vi "IMS Stepper V2.vi"() -> ()   [LabVIEW 2018]
doc: "Use this template to build a producer/consumer design pattern with events to produce queue items. Use this design pattern instead of the User Interface Event Handler pattern for user interfaces when you want to execute code asynchronously in response to an event without slowing the user interface responsiveness."
uses:
  stepper motor state.ctl
  stepper graphics internal event.ctl
  stepper graphics action.ctl
  stepper graphics internal state.ctl
  publisher action.ctl
  slider action.ctl
panel:
  in  "Tab Control":enum32{"main", "init&stuff", "ignore"}(tab)
  in  "stepper state":T1=enum."stopped"
  in  "set angle":dbl(slide)=-18.244680851063833 scale=-95.0..95.0 scale format="%^#6_6g"
  in  "XY Graph":cluster{dbl[], dbl[]}[](graph)=[{[-0.2849184585575504, -0.22366098996767705, -0.16240352137780373, -0.10114605278793037, -0.03988858419805705, 0.02136888439181628, 0.08262635298168963, 0.14388382157156293, 0.20514129016143628, 0.2663987587513096, 0.32765622734118294, 0.3889136959310563, 0.45017116452092965, 0.511428633110803, 0.5726861017006762, 0.6339435702905496, 0.695201038880423, 0.7564585074702963, 0.8177159760601695, 0.878973444650043], [0.09392269147117449, 0.07372931280487197, 0.053535934138569455, 0.03334255547226694, 0.013149176805964419, -0.007044201860338106, -0.027237580526640617, -0.04743095919294313, -0.06762433785924565, -0.08781771652554818, -0.1080110951918507, -0.1282044738581532, -0.14839785252445573, -0.16859123119075825, -0.18878460985706075, -0.2089779885233633, -0.2291713671896658, -0.2493647458559683, -0.26955812452227085, -0.28975150318857334]}, {[0.02614672282429747, 0.020525177417073513, 0.014903632009849559, 0.0092820866026256, 0.003660541195401646, -0.0019610042118223085, -0.00758254961904627, -0.013204095026270225, -0.01882564043349418, -0.024447185840718134, -0.03006873124794209, -0.03569027665516605, -0.04131182206239001, -0.04693336746961396, -0.05255491287683792, -0.05817645828406187, -0.06379800369128583, -0.06941954909850978, -0.07504109450573374, -0.08066263991295769], [0.2988584094275236, 0.23460385140060602, 0.17034929337368845, 0.10609473534677089, 0.04184017731985329, -0.022414380707064308, -0.08666893873398185, -0.15092349676089944, -0.21517805478781704, -0.27943261281473464, -0.34368717084165223, -0.40794172886856983, -0.4721962868954873, -0.5364508449224049, -0.6007054029493225, -0.6649599609762401, -0.7292145190031577, -0.7934690770300753, -0.8577236350569929, -0.9219781930839105]}, {[1.0, 0.9980267284282716, 0.9921147013144779, 0.9822872507286887, 0.9685831611286311, 0.9510565162951535, 0.9297764858882513, 0.9048270524660195, 0.8763066800438636, 0.8443279255020151, 0.8090169943749475, 0.7705132427757891, 0.7289686274214116, 0.6845471059286886, 0.6374239897486896, 0.587785252292473, 0.5358267949789965, 0.48175367410171516, 0.42577929156507266, 0.36812455268467786, 0.30901699437494745, 0.24868988716485474, 0.18738131458572452, 0.12533323356430426, 0.0627905195293133, -1.6081428723391245e-16, -0.0627905195293134, -0.12533323356430437, -0.18738131458572482, -0.24868988716485485, -0.30901699437494756, -0.368124552684678, -0.4257792915650727, -0.48175367410171543, -0.5358267949789969, -0.587785252292473, -0.6374239897486897, -0.6845471059286887, -0.7289686274214117, -0.7705132427757894, -0.8090169943749473, -0.8443279255020151, -0.8763066800438636, -0.9048270524660196, -0.9297764858882515, -0.9510565162951536, -0.9685831611286311, -0.9822872507286887, -0.9921147013144779, -0.9980267284282716, -1.0, -0.9980267284282716, -0.9921147013144779, -0.9822872507286886, -0.9685831611286311, -0.9510565162951535, -0.9297764858882512, -0.9048270524660195, -0.8763066800438635, -0.844327925502015, -0.8090169943749472, -0.770513242775789, -0.7289686274214116, -0.6845471059286886, -0.6374239897486895, -0.5877852522924732, -0.5358267949789963, -0.48175367410171527, -0.42577929156507216, -0.3681245526846778, -0.30901699437494756, -0.24868988716485443, -0.18738131458572463, -0.12533323356430373, -0.06279051952931321, -1.836909530733566e-16, 0.06279051952931372, 0.12533323356430423, 0.18738131458572513, 0.24868988716485493, 0.30901699437494723, 0.36812455268467825, 0.4257792915650726, 0.4817536741017157, 0.5358267949789968, 0.5877852522924737, 0.63742398974869, 0.6845471059286886, 0.7289686274214119, 0.7705132427757894, 0.8090169943749478, 0.8443279255020153, 0.8763066800438636, 0.9048270524660197, 0.9297764858882515, 0.9510565162951538, 0.9685831611286312, 0.9822872507286887, 0.9921147013144779, 0.9980267284282716], [0.0, 0.06279051952931337, 0.12533323356430426, 0.18738131458572463, 0.2486898871648548, 0.3090169943749474, 0.368124552684678, 0.4257792915650727, 0.4817536741017153, 0.5358267949789967, 0.5877852522924731, 0.6374239897486897, 0.6845471059286887, 0.7289686274214116, 0.7705132427757893, 0.8090169943749475, 0.8443279255020151, 0.8763066800438637, 0.9048270524660196, 0.9297764858882515, 0.9510565162951535, 0.9685831611286311, 0.9822872507286887, 0.9921147013144779, 0.9980267284282716, 1.0, 0.9980267284282716, 0.9921147013144778, 0.9822872507286886, 0.9685831611286311, 0.9510565162951535, 0.9297764858882513, 0.9048270524660195, 0.8763066800438635, 0.844327925502015, 0.8090169943749475, 0.7705132427757893, 0.7289686274214114, 0.6845471059286885, 0.6374239897486895, 0.5877852522924732, 0.5358267949789967, 0.4817536741017152, 0.4257792915650725, 0.36812455268467775, 0.3090169943749471, 0.24868988716485482, 0.18738131458572457, 0.1253332335643041, 0.06279051952931314, -3.216285744678249e-16, -0.06279051952931335, -0.12533323356430429, -0.18738131458572477, -0.24868988716485502, -0.30901699437494773, -0.3681245526846783, -0.42577929156507266, -0.4817536741017154, -0.5358267949789968, -0.5877852522924734, -0.63742398974869, -0.6845471059286887, -0.7289686274214116, -0.7705132427757894, -0.8090169943749473, -0.8443279255020153, -0.8763066800438636, -0.9048270524660198, -0.9297764858882515, -0.9510565162951535, -0.9685831611286312, -0.9822872507286887, -0.9921147013144779, -0.9980267284282716, -1.0, -0.9980267284282716, -0.9921147013144779, -0.9822872507286886, -0.9685831611286311, -0.9510565162951536, -0.9297764858882512, -0.9048270524660196, -0.8763066800438634, -0.844327925502015, -0.809016994374947, -0.770513242775789, -0.7289686274214116, -0.6845471059286883, -0.6374239897486896, -0.5877852522924726, -0.5358267949789963, -0.4817536741017153, -0.4257792915650722, -0.36812455268467786, -0.3090169943749468, -0.2486898871648545, -0.18738131458572468, -0.1253332335643038, -0.06279051952931326]}, {[0.1, 0.09980267284282716, 0.0992114701314478, 0.09822872507286888, 0.09685831611286311, 0.09510565162951536, 0.09297764858882514, 0.09048270524660196, 0.08763066800438636, 0.08443279255020152, 0.08090169943749476, 0.07705132427757892, 0.07289686274214116, 0.06845471059286887, 0.06374239897486897, 0.05877852522924731, 0.05358267949789966, 0.04817536741017152, 0.042577929156507266, 0.03681245526846779, 0.030901699437494747, 0.024868988716485477, 0.018738131458572452, 0.012533323356430426, 0.006279051952931331, -1.6081428723391246e-17, -0.0062790519529313405, -0.012533323356430438, -0.018738131458572484, -0.024868988716485487, -0.030901699437494757, -0.0368124552684678, -0.04257792915650727, -0.048175367410171546, -0.05358267949789969, -0.05877852522924731, -0.06374239897486898, -0.06845471059286888, -0.07289686274214117, -0.07705132427757894, -0.08090169943749474, -0.08443279255020152, -0.08763066800438636, -0.09048270524660196, -0.09297764858882515, -0.09510565162951537, -0.09685831611286311, -0.09822872507286888, -0.0992114701314478, -0.09980267284282716, -0.1, -0.09980267284282716, -0.0992114701314478, -0.09822872507286887, -0.09685831611286311, -0.09510565162951536, -0.09297764858882512, -0.09048270524660196, -0.08763066800438635, -0.0844327925502015, -0.08090169943749473, -0.07705132427757891, -0.07289686274214116, -0.06845471059286887, -0.06374239897486896, -0.05877852522924733, -0.05358267949789963, -0.04817536741017153, -0.04257792915650722, -0.036812455268467784, -0.030901699437494757, -0.024868988716485445, -0.018738131458572463, -0.012533323356430374, -0.006279051952931321, -1.836909530733566e-17, 0.006279051952931373, 0.012533323356430424, 0.018738131458572515, 0.024868988716485494, 0.030901699437494726, 0.036812455268467825, 0.042577929156507266, 0.048175367410171574, 0.05358267949789968, 0.05877852522924737, 0.063742398974869, 0.06845471059286887, 0.07289686274214119, 0.07705132427757894, 0.08090169943749478, 0.08443279255020153, 0.08763066800438636, 0.09048270524660197, 0.09297764858882515, 0.09510565162951538, 0.09685831611286312, 0.09822872507286888, 0.0992114701314478, 0.09980267284282716], [0.0, 0.006279051952931338, 0.012533323356430426, 0.018738131458572463, 0.02486898871648548, 0.03090169943749474, 0.0368124552684678, 0.04257792915650727, 0.04817536741017153, 0.05358267949789967, 0.058778525229247314, 0.06374239897486898, 0.06845471059286888, 0.07289686274214116, 0.07705132427757894, 0.08090169943749476, 0.08443279255020152, 0.08763066800438638, 0.09048270524660196, 0.09297764858882515, 0.09510565162951536, 0.09685831611286311, 0.09822872507286888, 0.0992114701314478, 0.09980267284282716, 0.1, 0.09980267284282716, 0.09921147013144778, 0.09822872507286887, 0.09685831611286311, 0.09510565162951536, 0.09297764858882514, 0.09048270524660196, 0.08763066800438635, 0.0844327925502015, 0.08090169943749476, 0.07705132427757894, 0.07289686274214115, 0.06845471059286885, 0.06374239897486896, 0.05877852522924733, 0.05358267949789967, 0.048175367410171525, 0.04257792915650725, 0.03681245526846778, 0.030901699437494712, 0.024868988716485484, 0.01873813145857246, 0.01253332335643041, 0.0062790519529313145, -3.216285744678249e-17, -0.006279051952931335, -0.01253332335643043, -0.018738131458572477, -0.024868988716485504, -0.030901699437494774, -0.03681245526846783, -0.042577929156507266, -0.04817536741017154, -0.05358267949789968, -0.05877852522924734, -0.063742398974869, -0.06845471059286888, -0.07289686274214116, -0.07705132427757894, -0.08090169943749474, -0.08443279255020153, -0.08763066800438636, -0.09048270524660199, -0.09297764858882515, -0.09510565162951536, -0.09685831611286312, -0.09822872507286888, -0.0992114701314478, -0.09980267284282716, -0.1, -0.09980267284282716, -0.0992114701314478, -0.09822872507286887, -0.09685831611286311, -0.09510565162951537, -0.09297764858882512, -0.09048270524660196, -0.08763066800438635, -0.0844327925502015, -0.0809016994374947, -0.07705132427757891, -0.07289686274214116, -0.06845471059286883, -0.06374239897486897, -0.05877852522924726, -0.05358267949789963, -0.04817536741017153, -0.042577929156507224, -0.03681245526846779, -0.03090169943749468, -0.02486898871648545, -0.01873813145857247, -0.012533323356430379, -0.006279051952931327]}, {[0.0, 0.0, 0.0, 0.0, 0.0, 0.0, 0.0, 0.0, 0.0, 0.0, 0.0, 0.0, 0.0, 0.0, 0.0, 0.0, 0.0, 0.0, 0.0, 0.0], [1.1, 1.135, 1.1700000000000002, 1.205, 1.24, 1.2750000000000001, 1.31, 1.345, 1.3800000000000001, 1.415, 1.4500000000000002, 1.485, 1.52, 1.5550000000000002, 1.59, 1.625, 1.6600000000000001, 1.695, 1.73, 1.7650000000000001]}, {[6.735334946023075e-17, 6.796565263714194e-17, 6.857795581405312e-17, 6.919025899096432e-17, 6.980256216787551e-17, 7.04148653447867e-17, 7.102716852169788e-17, 7.163947169860908e-17, 7.225177487552027e-17, 7.286407805243145e-17, 7.347638122934264e-17, 7.408868440625383e-17, 7.470098758316503e-17, 7.53132907600762e-17, 7.59255939369874e-17, 7.653789711389858e-17, 7.715020029080977e-17, 7.776250346772096e-17, 7.837480664463216e-17, 7.898710982154334e-17], [1.1, 1.11, 1.12, 1.1300000000000001, 1.1400000000000001, 1.1500000000000001, 1.1600000000000001, 1.1700000000000002, 1.1800000000000002, 1.1900000000000002, 1.2000000000000002, 1.21, 1.22, 1.23, 1.24, 1.25, 1.26, 1.27, 1.28, 1.29]}, {[-0.09587131702242406, -0.09674287444990064, -0.09761443187737723, -0.0984859893048538, -0.0993575467323304, -0.10022910415980697, -0.10110066158728355, -0.10197221901476014, -0.10284377644223672, -0.10371533386971331, -0.10458689129718989, -0.10545844872466646, -0.10633000615214305, -0.10720156357961963, -0.10807312100709622, -0.1089446784345728, -0.10981623586204937, -0.11068779328952597, -0.11155935071700254, -0.11243090814447912], [-1.0958141679009201, -1.1057761148818375, -1.115738061862755, -1.1257000088436726, -1.13566195582459, -1.1456239028055073, -1.1555858497864249, -1.1655477967673424, -1.1755097437482598, -1.1854716907291771, -1.1954336377100947, -1.2053955846910123, -1.2153575316719296, -1.225319478652847, -1.2352814256337645, -1.245243372614682, -1.2552053195955994, -1.2651672665765168, -1.2751292135574344, -1.285091160538352]}]
  out "cur angle":dbl(slide)=-95.0 scale=-95.0..95.0 scale format="%^#6_6g"
  in  "set step !":dbl(slide)=6845.744680851064 min=0.0 max=16000.0 scale=0.0..16500.0 scale format="%^#6_6g"
  out "cur step":dbl(slide) scale=0.0..16500.0
  in  "Go!":bool
  in  "Stop!":bool
  in  "set speed!":i32=2500
  out "Moving..":bool
  out "error out":errorcluster
  out "Current Bottom Position":dbl format="%.4f"
  in  "Move to Bottom Position (deg or in)":dbl=95.83933701824397 format="%.4f"
  in  "Rotator":T2(ring)=enum."System B 50 mm Magnet"
  out "Timeout error":bool
  in  "Exit!":bool
  in  "Instrument Address":refnum<visa-resource-name>="ASRL2::INSTR"
  in  "Set to zero!":bool
  in  "Init!":bool
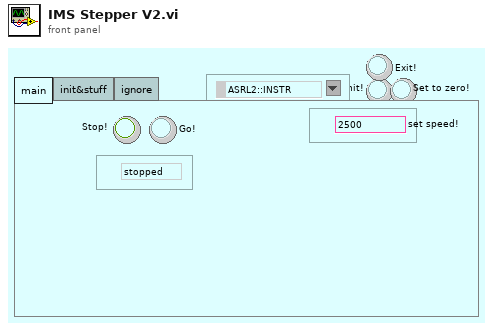
[diagram p1: front panel]
types:
  T1 = typedef "stepper motor state.ctl" = enum16{"moving", "stopped"}
  T2 = enum16{"Dilution Fridge SCM 1", "System A SCM 2", "System B 50 mm Magnet", "He-3 32 mm Magnet", "Portable Dil Fridge Rotator", "Linear Position", "System E Probe 1"}
  T3 = typedef "stepper graphics internal state.ctl" = cluster{"set pos slider":refnum<vi>, "cur angle slider":refnum<vi>, "XY Graph":refnum<vi>, "set angle":dbl, "current angle":dbl, "set angle slider":refnum<vi>, "current pos... slider":refnum<vi>, "current pos":dbl, "set pos":dbl}
  T4 = typedef "stepper graphics action.ctl" = enum16{"--update circle", "set step slider moves", "cursor moves", "current pos changed", "init", "void", "--draw current lie", "--draw set line", "--move current step slider", "--move set step slider", "--draw limit lines", "check", "--move set angle slider", "--move current angle slider", "set angle slider moves", "--move cursor", "set set step", "set current step", "read"}
  T5 = typedef "stepper graphics internal event.ctl" = enum16{"set slider moves", "update scale", "exit", "current positon changed", "stop", "go", "set speed", "set to zero", "sync"}
  T6 = typedef "slider action.ctl" = enum16{"check", "copy range", "set from value", "set from ratio", "set from slider", "read using other slider"}
  T7 = typedef "publisher action.ctl" = enum16{"set", "get"}
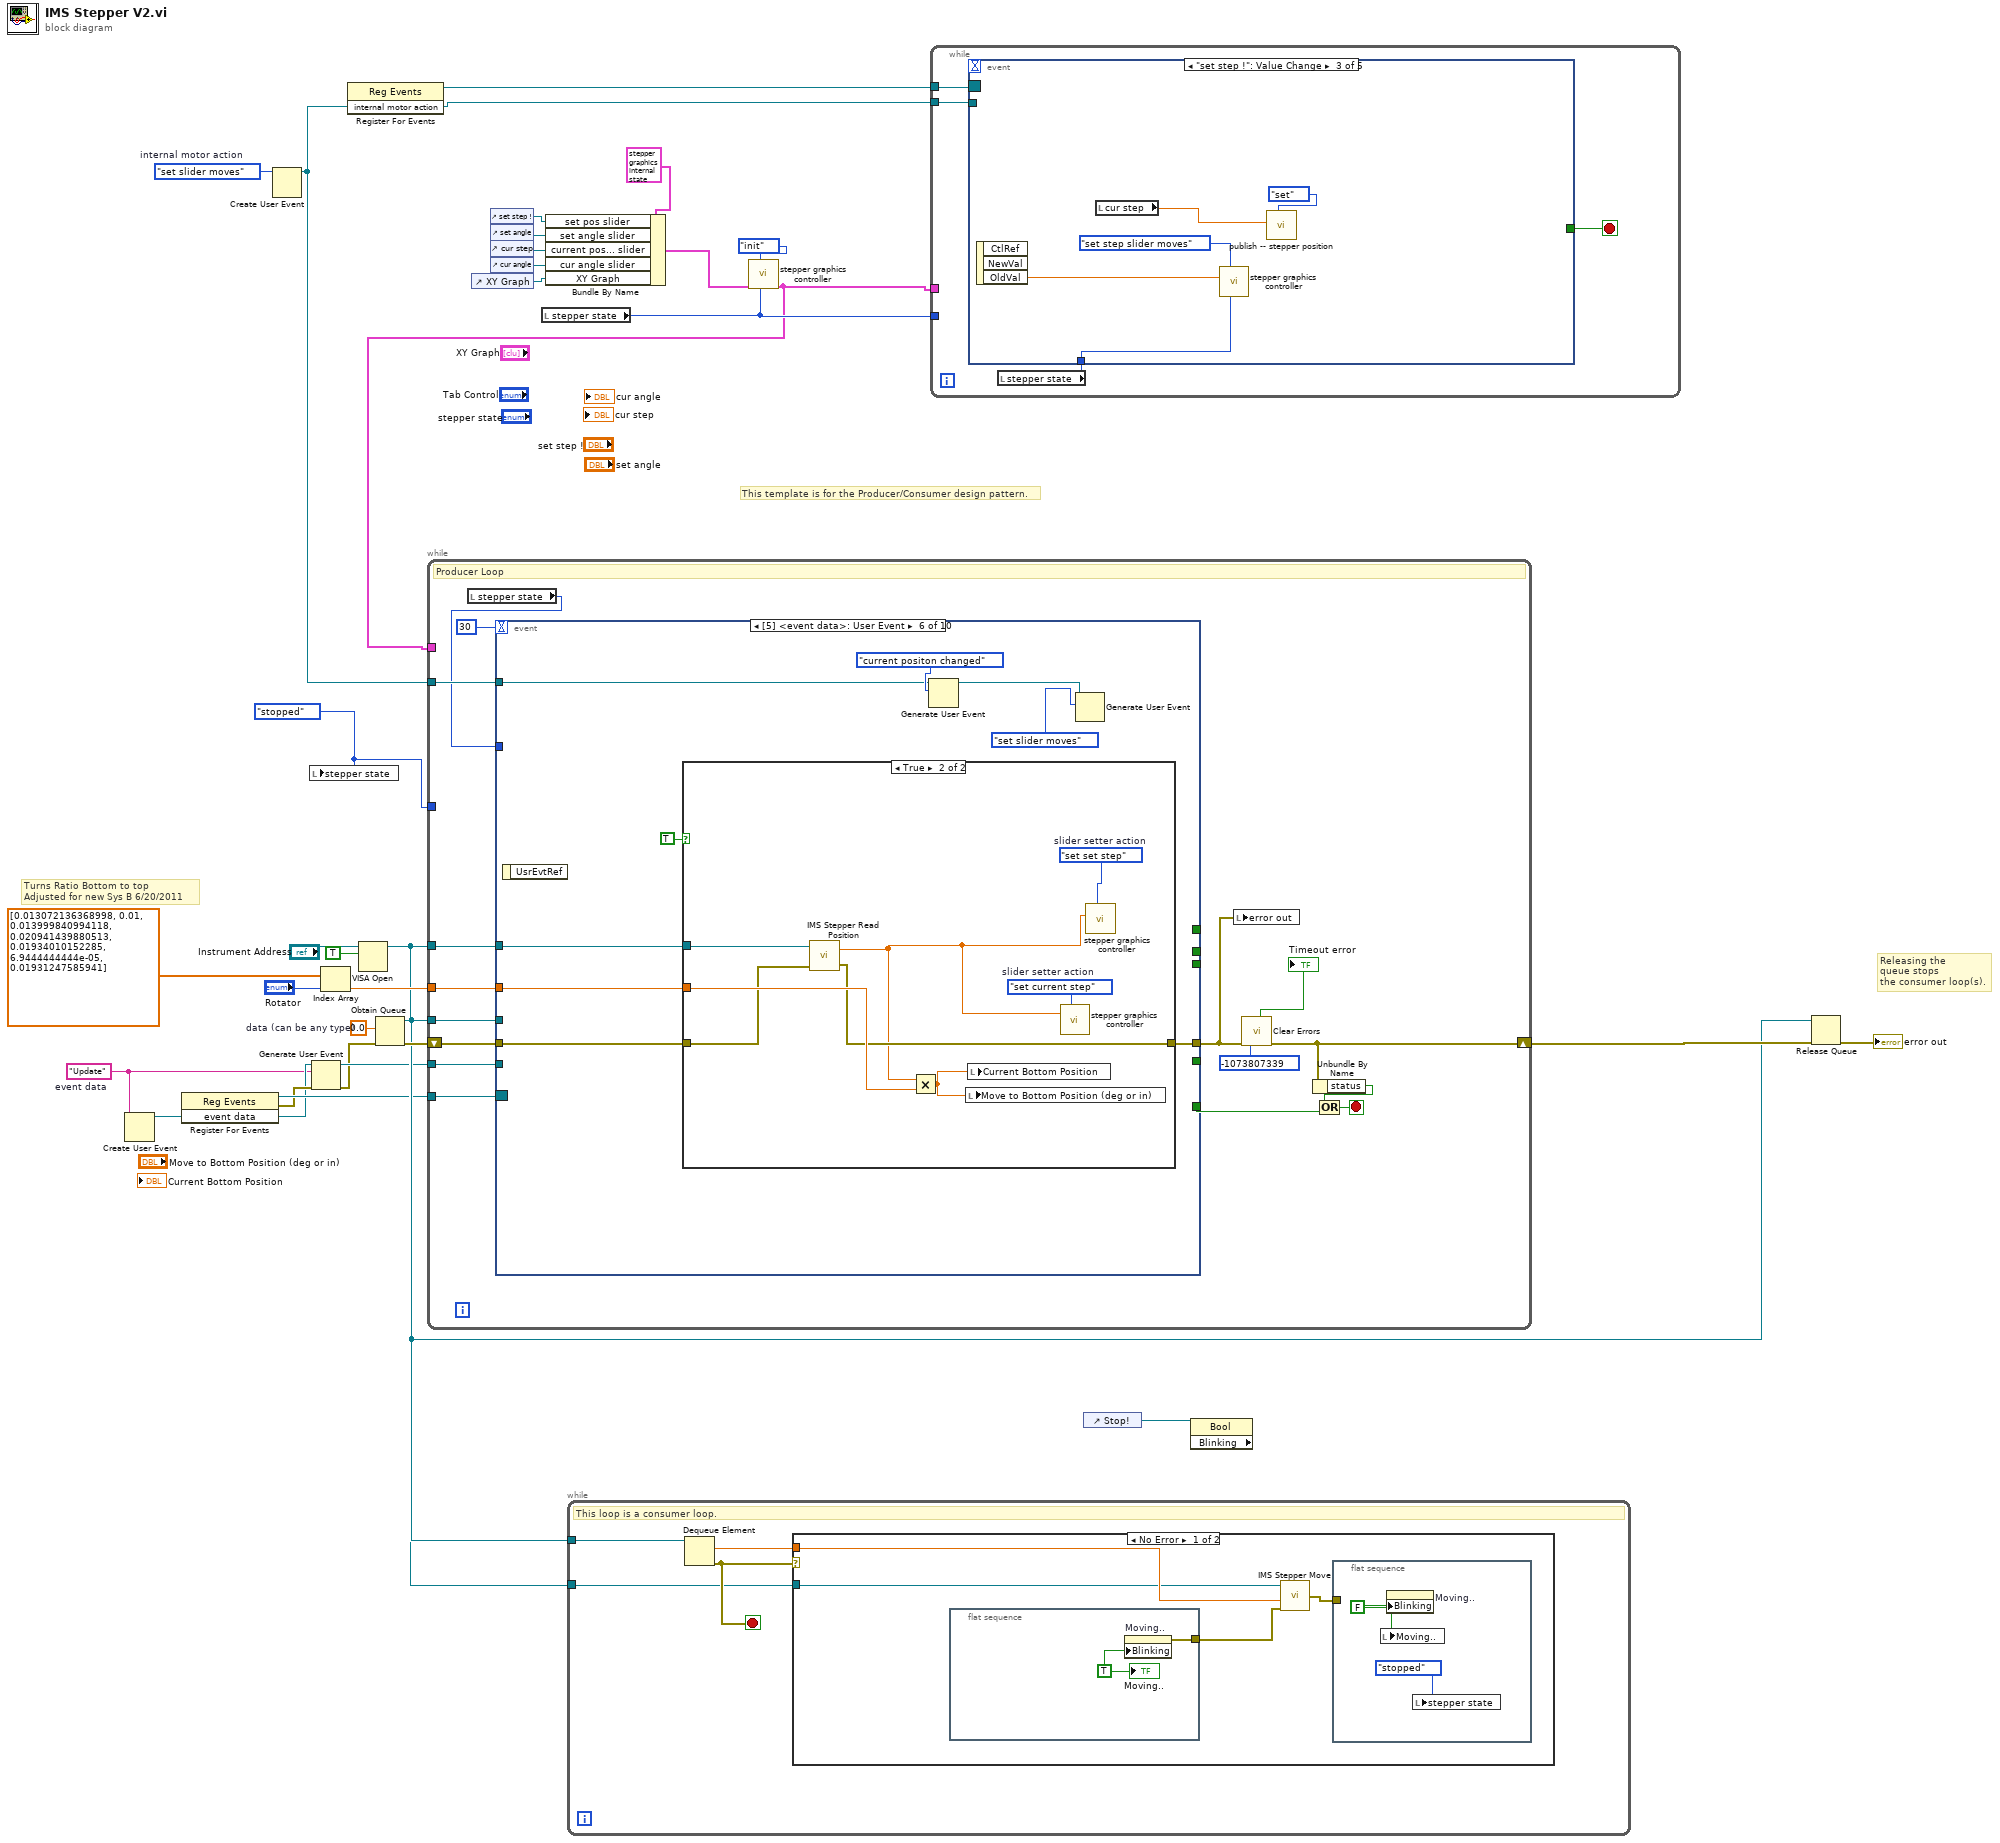
[diagram p0: block diagram]
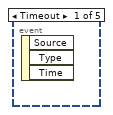
[diagram p2: hidden frame]
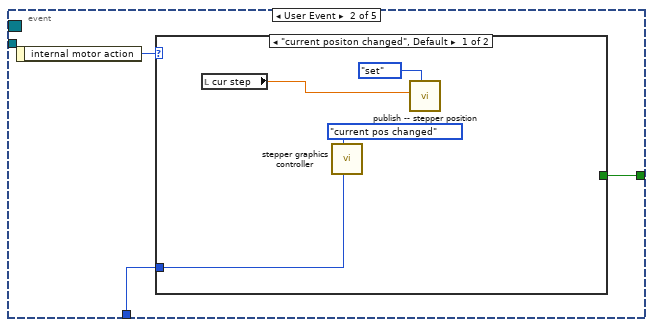
[diagram p3: hidden frame]
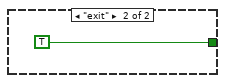
[diagram p4: hidden frame]
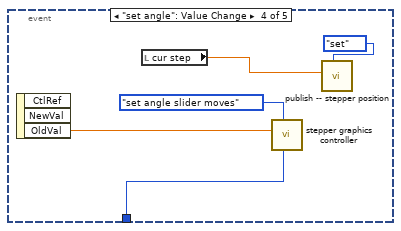
[diagram p5: hidden frame]
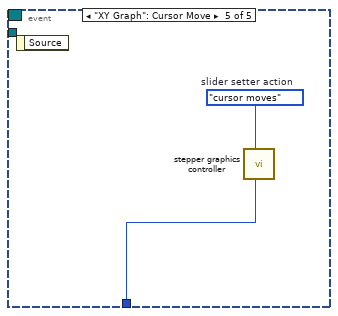
[diagram p6: hidden frame]
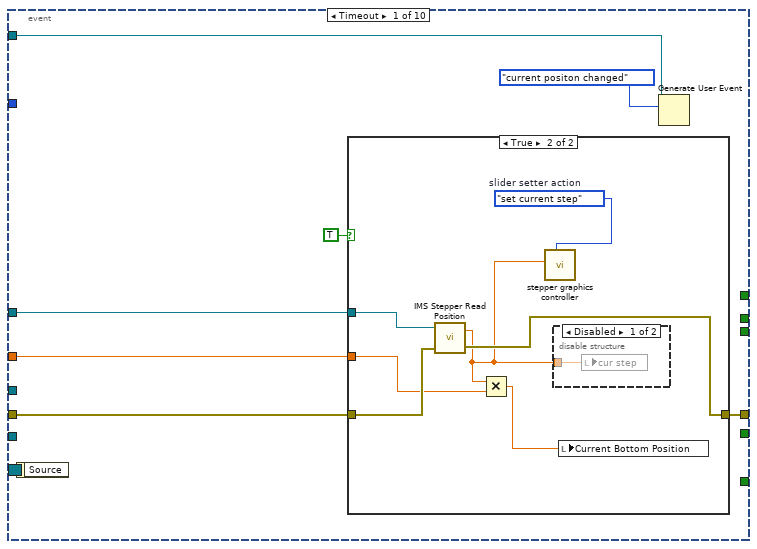
[diagram p8: hidden frame]
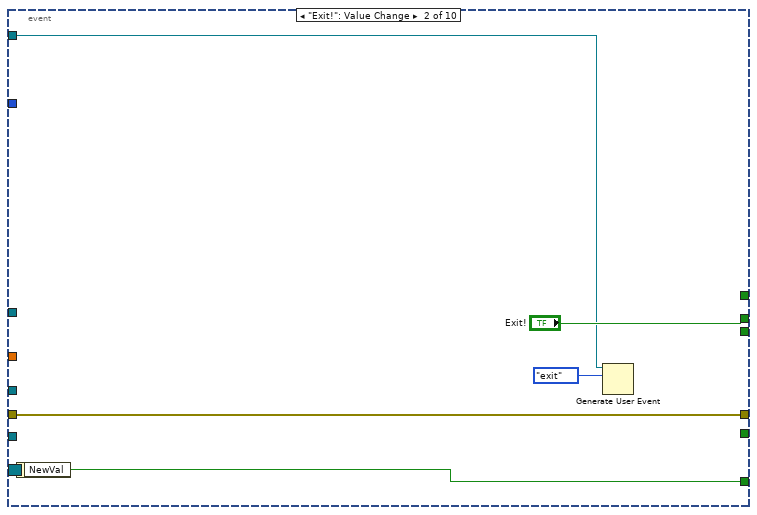
[diagram p11: hidden frame]
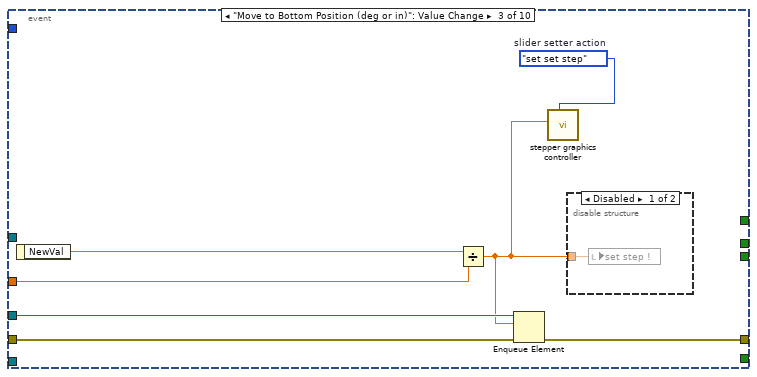
[diagram p12: hidden frame]
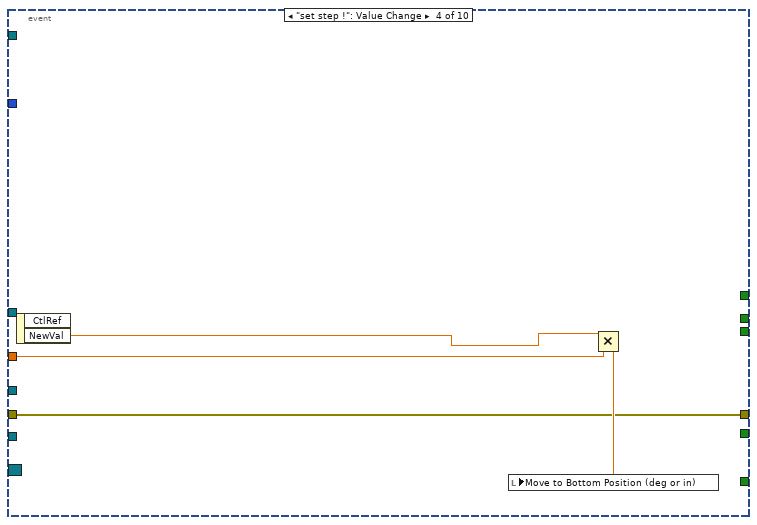
[diagram p14: hidden frame]
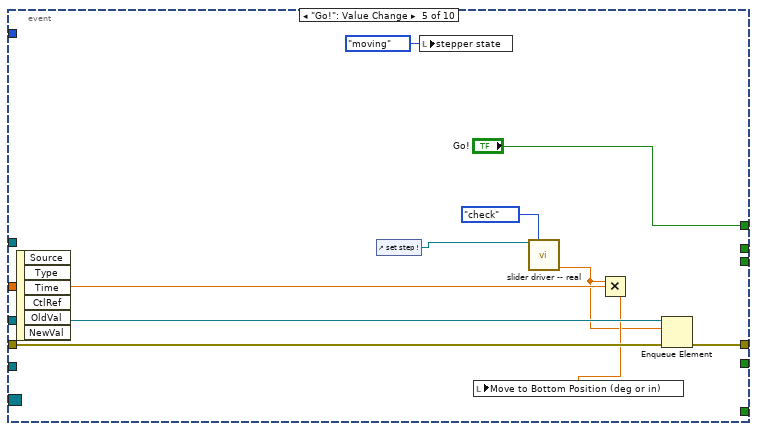
[diagram p15: hidden frame]
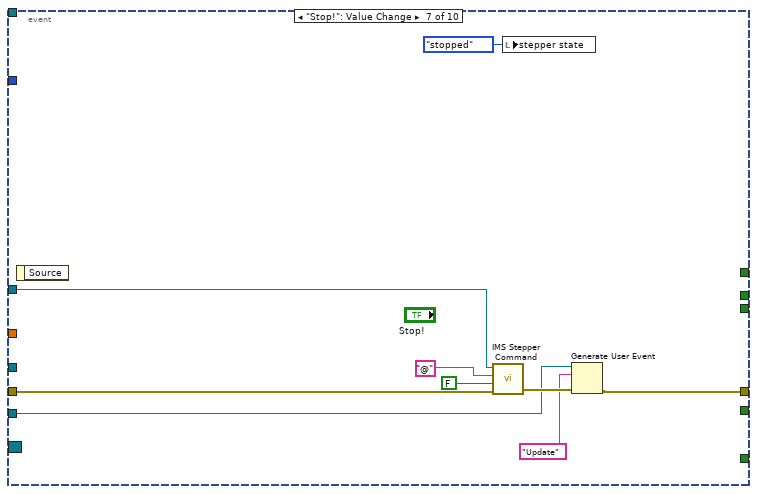
[diagram p17: hidden frame]
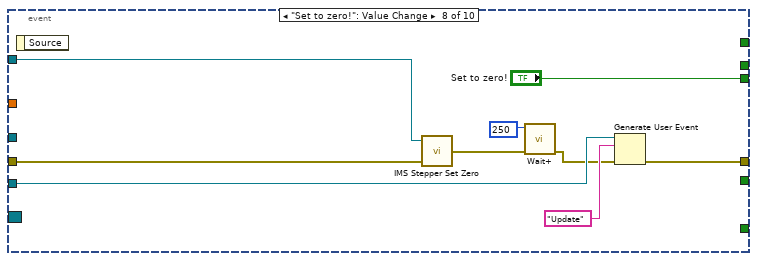
[diagram p18: hidden frame]
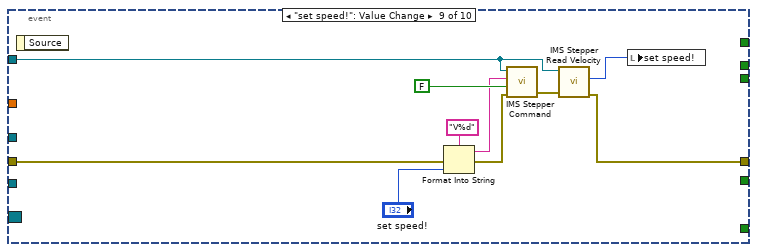
[diagram p19: hidden frame]
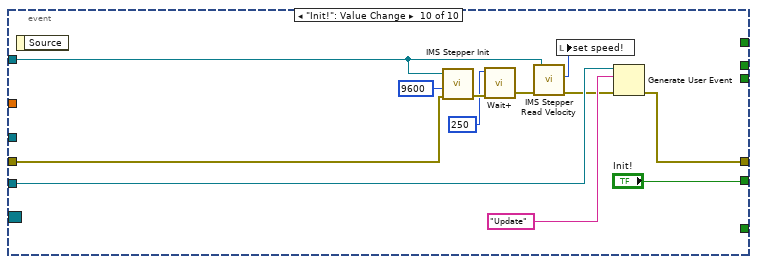
[diagram p20: hidden frame]
diagram:
  w3 = stepper_motor_state."stopped" ("stepper state")
  w14 = stepper_graphics_internal_event."set slider moves"  # internal motor action
  w17 = "Update"  # event data
  w30 = 0.0  # data (can be any type)
  # "Turns Ratio Bottom to top\nAdjusted for new Sys B 6/20/2011"
  # "Releasing the\nqueue stops\nthe consumer loop(s)."
  # "This template is for the Producer/Consumer design pattern."
  n1 = Create User Event(user event datatype=w17) -> (user event=w20:refnum<user-event>)  [unwired: 1 in, 1 out]
  n2 = register-events(w20) -> (reference out=w22:refnum<event-registration>, error out=w21:errorcluster)  [unwired: 2 in]
  n3 = Create User Event(user event datatype=w14) -> (user event=w11:refnum<user-event>)  [unwired: 1 in, 1 out]
  n4 = local write "stepper state"(w3) -> ()
  n5 = Generate User Event(user event=w20, event data cluster=w17, error in=w21) -> (user event out=w19:refnum<user-event>, error out=w18:errorcluster)  [unwired: 1 in]
  n6 = Index Array(array=dbl[] [0.013072136368998, 0.01, 0.013999840994118, 0.020941439880513, 0.01934010152285, 6.9444444444e-05, 0.01931247585941], index="Rotator") -> (element=w24:dbl)
  n7 = register-events(w11) -> (reference out=w15:refnum<event-registration>)  [unwired: 2 in, 1 out]
  n8 = VISA Open(duplicate session (F)=TRUE, VISA resource name="Instrument Address") -> (VISA resource name=w23:refnum<visa-resource-name>)  [unwired: 3 in, 1 out]
  n9 = Obtain Queue(element data type=w30, error in (no error)=w18) -> (queue out=w29:refnum<queue>, error out=w32:errorcluster)  [unwired: 3 in, 1 out]
  n10 = control-ref of="XY Graph"() -> (w10:refnum<vi>)
  n11 = control-ref of="set step !"() -> (w6:refnum<vi>)
  n12 = control-ref of="set angle"() -> (w7:refnum<vi>)
  n13 = control-ref of="cur step"() -> (w8:refnum<vi>)
  n14 = control-ref of="cur angle"() -> (w9:refnum<vi>)
  n15 = local read "stepper state"() -> (w12:T1)
  n16 = Bundle By Name(cluster=T3 {"set pos slider"=refnum, "cur angle slider"=refnum, "XY Graph"=refnum, "set angle"=0.0, "current angle"=0.0, "set angle slider"=refnum, "current pos... slider"=refnum, "current pos"=0.0, "set pos"=0.0} ("stepper graphics internal state"), "set pos slider"=w6, "set angle slider"=w7, "current pos... slider"=w8, "cur angle slider"=w9, "XY Graph"=w10) -> (w5:T3)
  n17 = while {
    tunnel: w29 -> [w36]
    tunnel: w23 -> [w33]
    stop <- w35 stop-if-true
    # "This loop is a consumer loop."
    n18 = Dequeue Element(queue=w36) -> (element=w34:dbl, error out=w35:errorcluster)  [unwired: 2 in, 2 out]
    n19 = case shown="No Error" w35 {
      tunnel: w34 -> [w40 _]
      tunnel: w33 -> [w39 _]
      frame No Error {
        n20 = flat-sequence {
          tunnel: [w41] -> w38
          frame #0 {
            w42 = TRUE ("Moving")
            n21 = property on="Moving.." class="Bool (strict)"("Blinking"=w42) -> (error out=w41:errorcluster)  [unwired: 2 in, 1 out]
            "Moving.." <- w42
          }
        }
        n22 = call "IMS Stepper Move.vi"("Instrument Address"=w39, "Distance"=w40, "error in (no error)"=w38) -> ("error out"=w37:errorcluster)  [unwired: 2 in]
        n23 = flat-sequence {
          tunnel: w37 -> [_]
          frame #0 {
            w44 = FALSE ("Moving")
            n24 = local write "Moving.."(w44) -> ()
            n25 = property on="Moving.." class="Bool (strict)"("Blinking"=w44) -> ()  [unwired: 2 in, 2 out]
            n26 = local write "stepper state"(stepper_motor_state."stopped" ("stepper state")) -> ()
          }
        }
      }
      frame Error {
      }
    }
  }
  n27 = call "stepper graphics controller.vi"("stepper motor state"=w12, "stepper graphics action"=stepper_graphics_action."init" ("slider setter action"), "stepper graphics internal state"=w5) -> ("stepper graphics internal state OUT"=w4:T3)  [unwired: 7 in, 1 out]
  n28 = while {
    shift-right: [w48] -> w31
    shift-left: w32 -> [w59]
    tunnel: w29 -> [w60]
    tunnel: w23 -> [w54]
    tunnel: w24 -> [w53]
    tunnel: w22 -> [w52]
    tunnel: w19 -> [w51]
    tunnel: w11 -> [w46]
    tunnel: w4 -> [_]
    tunnel: w3 -> [_]
    stop <- w57 stop-if-true
    # "Producer Loop"
    n29 = local read "stepper state"() -> (w45:T1)
    n30 = event shown="[5] <event data>: User Event" {
      selector: w52 -> [_ _ _ _ _ _ _ _ _ _]
      dyn-events: _ -> [_ _ _ _ _ _ _ _ _ _]
      timeout: 30 -> [_ _ _ _ _ _ _ _ _ _]
      tunnel: w60 -> [_ _ w88 _ w104 _ _ _ _ _]
      tunnel: w59 -> [w67 w81 w87 w92 w103 w111 w129 w140 w146 w159]
      tunnel: [w62 w81 w86 w92 w102 w108 w127 w138 w141 w162] -> w47
      tunnel: [_ w80 _ _ _ _ _ _ _ _] -> w58
      tunnel: w54 -> [w66 _ _ _ _ w112 w131 w139 w143 w156]
      tunnel: w53 -> [w65 _ w85 w94 w101 w113 _ _ _ _]
      tunnel: w51 -> [_ _ _ _ _ _ w125 w137 _ w161]
      tunnel: [_ _ _ _ _ _ _ "Set to zero!" _ _] -> _
      tunnel: [_ _ _ _ _ _ _ _ _ "Init!"] -> _
      tunnel: [_ "Exit!" _ _ _ _ _ _ _ _] -> _
      tunnel: w46 -> [w64 w77 _ w91 _ w109 _ _ _ _]
      tunnel: [_ _ _ _ "Go!" _ _ _ _ _] -> _
      tunnel: [_ _ _ w91 _ _ _ _ _ _] -> _
      tunnel: w45 -> [_ _ _ _ _ _ _ _ _ _]
      event Timeout {
        n31 = event-data() -> ()  [unwired: 1 in, 1 out]
        n32 = case shown="True" TRUE {
          tunnel: w67 -> [w68 w75]
          tunnel: w66 -> [_ w74]
          tunnel: w65 -> [_ w73]
          tunnel: [w68 w71] -> w62
          frame False {
          }
          frame True {
            w69 = stepper_graphics_action."set current step"  # slider setter action
            n33 = call "IMS Stepper Read Position.vi"("error in (no error)"=w75, "Instrument Address"=w74) -> ("error out"=w71:errorcluster, "Response"=w70:dbl)  [unwired: 1 in]
            n34 = Multiply(x=w70, y=w73) -> (x*y=w72:dbl)
            n35 = call "stepper graphics controller.vi"("stepper graphics action"=w69, "value"=w70) -> ()  [unwired: 8 in, 2 out]
            n36 = disable-structure shown="Disabled" {
              disable-tunnel: w70 -> [w76 _]
              frame Disabled {
                n37 = local write "cur step"(w76) -> ()
              }
              frame Enabled {
              }
            }
            n38 = local write "Current Bottom Position"(w72) -> ()
          }
        }
        n39 = Generate User Event(user event=w64, event data cluster=stepper_graphics_internal_event."current positon changed" ("event data")) -> ()  [unwired: 2 in, 2 out]
      }
      event "Exit!": Value Change {
        n40 = event-data() -> ("NewVal"=w80:bool)  [unwired: 1 in]
        n41 = Generate User Event(user event=w77, event data cluster=stepper_graphics_internal_event."exit" ("event data")) -> ()  [unwired: 2 in, 2 out]
      }
      event "Move to Bottom Position (deg or in)": Value Change {
        w82 = stepper_graphics_action."set set step"  # slider setter action
        n42 = event-data() -> ("NewVal"=w84:dbl)  [unwired: 1 in]
        n43 = Divide(x=w84, y=w85) -> (x/y=w83:dbl)
        n44 = Enqueue Element(queue=w88, element=w83, error in (no error)=w87) -> (error out=w86:errorcluster)  [unwired: 1 in, 2 out]
        n45 = call "stepper graphics controller.vi"("stepper graphics action"=w82, "value"=w83) -> ()  [unwired: 8 in, 2 out]
        n46 = disable-structure shown="Disabled" {
          disable-tunnel: w83 -> [w89 _]
          frame Disabled {
            n47 = local write "set step !"(w89) -> ()
          }
          frame Enabled {
          }
        }
      }
      event "set step !": Value Change {
        n48 = event-data() -> ("NewVal"=w90:dbl)  [unwired: 1 in, 1 out]
        n49 = Multiply(x=w90, y=w94) -> (x*y=w93:dbl)
        n50 = local write "Move to Bottom Position (deg or in)"(w93) -> ()
      }
      event "Go!": Value Change {
        n51 = event-data() -> ()  [unwired: 1 in, 6 out]
        n52 = control-ref of="set step !"() -> (w96:refnum<vi>)
        n53 = local write "stepper state"(stepper_motor_state."moving" ("stepper state")) -> ()
        n54 = call "slider driver -- real.vi"("slider in"=w96, "slider action"=slider_action."check") -> ("value OUT"=w98:dbl)  [unwired: 9 in, 4 out]
        n55 = Multiply(x=w98, y=w101) -> (x*y=w100:dbl)
        n56 = local write "Move to Bottom Position (deg or in)"(w100) -> ()
        n57 = Enqueue Element(queue=w104, element=w98, error in (no error)=w103) -> (error out=w102:errorcluster)  [unwired: 1 in, 2 out]
      }
      event User Event {
        n58 = event-data() -> ()  [unwired: 1 in, 1 out]
        n59 = case shown="True" TRUE {
          tunnel: w113 -> [_ w122]
          tunnel: w112 -> [_ w121]
          tunnel: w111 -> [w114 w120]
          tunnel: [w114 w118] -> w108
          frame False {
          }
          frame True {
            w116 = stepper_graphics_action."set current step"  # slider setter action
            w117 = stepper_graphics_action."set set step"  # slider setter action
            n60 = call "IMS Stepper Read Position.vi"("error in (no error)"=w120, "Instrument Address"=w121) -> ("error out"=w118:errorcluster, "Response"=w115:dbl)  [unwired: 1 in]
            n61 = Multiply(x=w115, y=w122) -> (x*y=w119:dbl)
            n62 = local write "Move to Bottom Position (deg or in)"(w119) -> ()
            n63 = local write "Current Bottom Position"(w119) -> ()
            n64 = call "stepper graphics controller.vi"("stepper graphics action"=w116, "value"=w115) -> ()  [unwired: 8 in, 2 out]
            n65 = call "stepper graphics controller.vi"("stepper graphics action"=w117, "value"=w115) -> ()  [unwired: 8 in, 2 out]
          }
        }
        n66 = Generate User Event(user event=w109, event data cluster=stepper_graphics_internal_event."current positon changed" ("event data")) -> (user event out=w107:refnum<user-event>)  [unwired: 2 in, 1 out]
        n67 = Generate User Event(user event=w107, event data cluster=stepper_graphics_internal_event."set slider moves" ("event data")) -> ()  [unwired: 2 in, 2 out]
      }
      event "Stop!": Value Change {
        n68 = event-data() -> ()  [unwired: 1 in, 1 out]
        n69 = call "IMS Stepper Command.vi"("Instrument Address"=w131, "Command"="@", "Mode"=FALSE, "error in (no error)"=w129) -> ("error out"=w126:errorcluster)  [unwired: 2 in, 2 out]
        n70 = local write "stepper state"(stepper_motor_state."stopped" ("stepper state")) -> ()
        n71 = Generate User Event(user event=w125, event data cluster="Update" ("event data"), error in=w126) -> (error out=w127:errorcluster)  [unwired: 1 in, 1 out]
      }
      event "Set to zero!": Value Change {
        n72 = event-data() -> ()  [unwired: 1 in, 1 out]
        n73 = call "IMS Stepper Set Zero.vi"("error in (no error)"=w140, "Instrument Address"=w139) -> ("error out"=w134:errorcluster)  [unwired: 1 in]
        n74 = call "Wait+.vi"("Error In"=w134, "milliseconds to wait"=u32 250) -> ("Error Out"=w133:errorcluster)  [unwired: 4 in, 1 out]
        n75 = Generate User Event(user event=w137, event data cluster="Update" ("event data"), error in=w133) -> (error out=w138:errorcluster)  [unwired: 1 in, 1 out]
      }
      event "set speed!": Value Change {
        n76 = event-data() -> ()  [unwired: 1 in, 1 out]
        n77 = Format Into String(format string="V%d", error in=w146, "set speed!") -> (resulting string=w147:string, error out=w145:errorcluster)  [unwired: 1 in]
        n78 = call "IMS Stepper Command.vi"("Instrument Address"=w143, "Command"=w147, "Mode"=FALSE, "error in (no error)"=w145) -> ("error out"=w144:errorcluster)  [unwired: 2 in, 2 out]
        n79 = call "IMS Stepper Read Velocity.vi"("error in (no error)"=w144, "Instrument Address"=w143) -> ("error out"=w141:errorcluster, "Velocity"=w142:i32)  [unwired: 3 in, 1 out]
        n80 = local write "set speed!"(w142) -> ()
      }
      event "Init!": Value Change {
        n81 = event-data() -> ()  [unwired: 1 in, 1 out]
        n82 = call "IMS Stepper Init.vi"("error in (no error)"=w159, "Baud Rate"=u32 9600, "Instrument Address"=w156) -> ("error out"=w153:errorcluster)  [unwired: 1 in, 1 out]
        n83 = call "Wait+.vi"("Error In"=w153, "milliseconds to wait"=u32 250) -> ("Error Out"=w154:errorcluster)  [unwired: 4 in, 1 out]
        n84 = call "IMS Stepper Read Velocity.vi"("error in (no error)"=w154, "Instrument Address"=w156) -> ("error out"=w157:errorcluster, "Velocity"=w155:i32)  [unwired: 3 in, 1 out]
        n85 = local write "set speed!"(w155) -> ()
        n86 = Generate User Event(user event=w161, event data cluster="Update" ("event data"), error in=w157) -> (error out=w162:errorcluster)  [unwired: 1 in, 1 out]
      }
    }
    n87 = local write "error out"(w47) -> ()
    n88 = call <vilib>:"Clear Errors.vi"("error in (no error)"=w47, "specific error code to clear (0: all)"=-1073807339) -> ("error out"=w48:errorcluster, "specific error cleared?"=→"Timeout error":bool)  [unwired: 4 in]
    n89 = Unbundle By Name(w48) -> ("status"=w56:bool)
    n90 = Or(x=w56, y=w58) -> (x .or. y?=w57:bool)
  }
  n91 = while {
    tunnel: w15 -> [w166]
    tunnel: w12 -> [_]
    tunnel: w11 -> [w164]
    tunnel: w4 -> [_]
    stop <- w165 stop-if-true
    n92 = local read "stepper state"() -> (w163:T1)
    n93 = event shown="[2] \"set step !\": Value Change" {
      selector: w166 -> [_ _ _ _ _]
      dyn-events: _ -> [_ _ _ _ _]
      timeout: _ -> [_ _ _ _ _]
      tunnel: [_ w168 _ _ _] -> w165
      tunnel: w164 -> [_ _ _ _ _]
      tunnel: w163 -> [_ w167 w175 w180 w185]
      event Timeout {
        n94 = event-data() -> ()  [unwired: 1 in, 3 out]
      }
      event User Event {
        n95 = event-data() -> ("internal motor action"=w169:T5)  [unwired: 1 in]
        n96 = case shown="\"current positon changed\", Default" w169 {
          tunnel: [_ TRUE] -> w168
          tunnel: w167 -> [w170 _]
          frame "current positon changed", Default {
            n97 = local read "cur step"() -> (w172:dbl)
            n98 = call "stepper graphics controller.vi"("stepper motor state"=w170, "stepper graphics action"=stepper_graphics_action."current pos changed" ("slider setter action")) -> ()  [unwired: 8 in, 2 out]
            n99 = call "publish -- stepper position.vi"("publisher action"=publisher_action."set", "stepper pos IN"=w172) -> ()  [unwired: 9 in, 1 out]
          }
          frame "exit" {
          }
        }
      }
      event "set step !": Value Change {
        n100 = event-data() -> ("OldVal"=w177:dbl)  [unwired: 1 in, 2 out]
        n101 = local read "cur step"() -> (w179:dbl)
        n102 = call "stepper graphics controller.vi"("stepper motor state"=w175, "stepper graphics action"=stepper_graphics_action."set step slider moves" ("slider setter action"), "value"=w177) -> ()  [unwired: 7 in, 2 out]
        n103 = call "publish -- stepper position.vi"("publisher action"=publisher_action."set", "stepper pos IN"=w179) -> ()  [unwired: 9 in, 1 out]
      }
      event "set angle": Value Change {
        n104 = event-data() -> ("OldVal"=w182:dbl)  [unwired: 1 in, 2 out]
        n105 = local read "cur step"() -> (w184:dbl)
        n106 = call "stepper graphics controller.vi"("stepper motor state"=w180, "stepper graphics action"=stepper_graphics_action."set angle slider moves" ("slider setter action"), "value"=w182) -> ()  [unwired: 7 in, 2 out]
        n107 = call "publish -- stepper position.vi"("publisher action"=publisher_action."set", "stepper pos IN"=w184) -> ()  [unwired: 9 in, 1 out]
      }
      event "XY Graph": Cursor Move {
        w186 = stepper_graphics_action."cursor moves"  # slider setter action
        n108 = event-data() -> ()  [unwired: 1 in, 1 out]
        n109 = call "stepper graphics controller.vi"("stepper motor state"=w185, "stepper graphics action"=w186) -> ()  [unwired: 8 in, 2 out]
      }
    }
  }
  n110 = control-ref of="Stop!"() -> (w2:refnum<vi>)
  n111 = property class="Bool" props=["Blinking"](reference=w2) -> ()  [unwired: 1 in, 3 out]
  n112 = Release Queue(queue=w29, error in (no error)=w31) -> (error out=→"error out":errorcluster)  [unwired: 1 in, 2 out]
